vi "Send to All Active Connections.vi"(8 "error in (no error)":errorcluster, 9 "Data":variant, 10 "Message":string, 11 "Multiplexed Messenger In":refnum<data-value>) -> (0 "error out":errorcluster, 3 "Multiplexed Messenger Out":refnum<data-value>)   [LabVIEW 2019, in "Network Messenger.lvlib" / "Multiplexed Messenger.lvclass"]
uses:
  <vilib>/gpm_packages/@cs/Network-interface/Source/Network Messenger/Multiplexed Messenger/Multiplexed Messenger.lvclass
  <vilib>/gpm_packages/@cs/Network-interface/Source/Network Messenger/Multiplexed Messenger/Multiplexed Messenger.lvclass/Multiplexed Messenger.ctl
  <vilib>/gpm_packages/@cs/Network-interface/Source/Network Messenger/Synchronous Write Callback/Synchronous Write Callback.lvclass/Synchronous Write Callback.ctl
  <vilib>/gpm_packages/@cs/Network-interface/Source/Network Messenger/Types/Message Packet.ctl
  <vilib>/gpm_packages/@cs/Network-interface/Source/MessagingInterfaces/WriteRequest/WriteRequest.lvclass/WriteRequest.ctl
  <vilib>/gpm_packages/@cs/Network-interface/Source/PersistantConnectionHandler/PersistantConnectionHandler Messages/Execute Write Request Msg/Execute Write Request Msg.lvclass/Execute Write Request Msg.ctl
  <vilib>/ActorFramework/Message Enqueuer/Message Enqueuer.lvclass/Message Enqueuer.ctl
  <vilib>/ActorFramework/Message Enqueuer/Enqueue.vi
  <vilib>/gpm_packages/@cs/Network-interface/Source/Network Messenger/Synchronous Write Callback/Synchronous Write Callback.lvclass
  C:/Program Files/National Instruments/LabVIEW 2019/vi.lib/gpm_packages/@cs/Network-interface/Source/MessagingInterfaces/IWriteExecutionCallback/IWriteExecutionCallback.lvclass
  <vilib>/gpm_packages/@cs/Network-interface/Source/Network Messenger/ClusterMessagePacket/ClusterMessagePacket.lvclass
  C:/Program Files/National Instruments/LabVIEW 2019/vi.lib/gpm_packages/@cs/Network-interface/Source/MessagingInterfaces/IPacket/IPacket.lvclass
  <vilib>/gpm_packages/@cs/Network-interface/Source/PersistantConnectionHandler/PersistantConnectionHandler Messages/Execute Write Request Msg/Execute Write Request Msg.lvclass
  C:/Program Files/National Instruments/LabVIEW 2019/vi.lib/ActorFramework/Message/Message.lvclass
  <vilib>/ActorFramework/Message Priority Queue/Priority Enqueue.vi
  <vilib>/gpm_packages/@cs/Network-interface/Source/MessagingInterfaces/WriteRequest/WriteRequest.lvclass
  <vilib>/gpm_packages/@cs/Network-interface/Source/Network Messenger/Network Messenger.lvlib
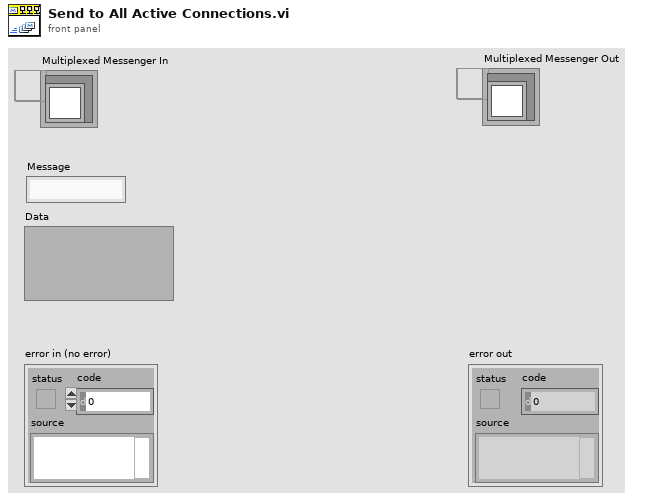
[diagram p1: front panel]
types:
  T1 = typedef "Network Messenger.lvlib/Message Packet.ctl" = cluster{"Msg":string, "Data":variant}
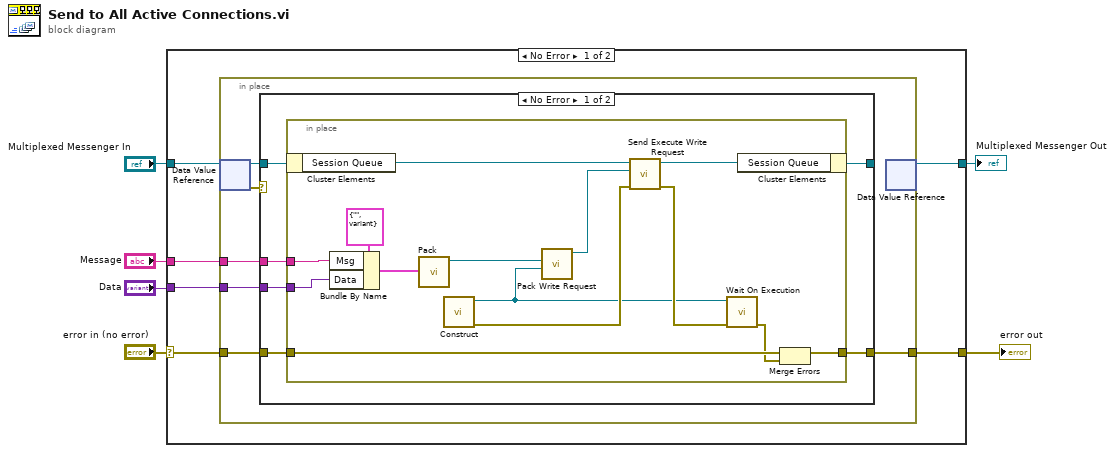
[diagram p0: block diagram]
diagram:
  n1 = case shown="No Error" "error in (no error)" {
    selector: "error in (no error)" -> [w10 w41]
    tunnel: "Multiplexed Messenger In" -> [w12 w42]
    tunnel: [w11 w42] -> w3
    tunnel: "Message" -> [w9 _]
    tunnel: "Data" -> [w8 _]
    tunnel: [w7 w41] -> w6
    frame No Error {
      n2 = in-place {
        in-place-border: w10 -> [w16]
        in-place-border: w9 -> [w14]
        in-place-border: w8 -> [w13]
        in-place-border: [w15] -> w7
        n3 = in-place-dvr #1(w12) -> (w18:refnum<class "Multiplexed Messenger.lvclass">, w17:errorcluster)
        n4 = case shown="No Error" w17 {
          selector: w17 -> [_ w39]
          tunnel: w18 -> [w24 w40]
          tunnel: [w23 w40] -> _
          tunnel: w16 -> [w22 _]
          tunnel: [w21 w39] -> w15
          tunnel: w14 -> [w20 _]
          tunnel: w13 -> [w19 _]
          frame No Error {
            n5 = in-place {
              in-place-border: w22 -> [w38]
              in-place-border: [w27] -> w21
              in-place-border: w20 -> [w33]
              in-place-border: w19 -> [w32]
              n6 = in-place-cluster #2(w24) -> ("Session Queue"=w37:refnum<class "Message Enqueuer.lvclass">)
              n7 = Bundle By Name(cluster=T1 {"Msg"="", "Data"=variant} ("Packet"), "Msg"=w33, "Data"=w32) -> (w34:T1)
              n8 = call <vilib>:"Pack.vi"("Packet"=w34) -> ("ClusterMessagePacket out"=w29:refnum<class "ClusterMessagePacket.lvclass">)  [unwired: 10 in]
              n9 = call <vilib>:"Construct.vi"() -> ("error out"=w28:errorcluster, "SynchronousWriteCallback out"=w25:refnum<class "Synchronous Write Callback.lvclass">)  [unwired: 10 in]
              n10 = call <vilib>:"Pack Write Request.vi"("Execution Callback"=w25, "Packet"=w29) -> ("WriteRequest out"=w31:refnum<class "WriteRequest.lvclass">)  [unwired: 9 in]
              n11 = call <vilib>:"Send Execute Write Request.vi"("error in (no error)"=w28, "Write Request"=w31, "Message Enqueuer"=w37) -> ("error out"=w30:errorcluster, "Message Enqueuer out"=w36:refnum<class "Message Enqueuer.lvclass">)  [unwired: 7 in]
              n12 = call <vilib>:"Wait On Execution.vi"("error in (no error)"=w30, "Synchronous Write Callback in"=w25) -> ("error out"=w26:errorcluster)  [unwired: 9 in]
              n13 = in-place-cluster #2("Session Queue"=w36) -> (w23:refnum<class "Multiplexed Messenger.lvclass">)
              n14 = Merge Errors(w38, w26) -> (w27:errorcluster)
            }
          }
          frame Error {
          }
        }
        n15 = in-place-dvr #1() -> (w11:refnum<data-value>)  [unwired: 1 in, 1 out]
      }
    }
    frame Error {
    }
  }
  "error out" <- w6
  "Multiplexed Messenger Out" <- w3
